vi "Set All Temp (SubVI).vi"(6 "Rate、speed":dbl, 9 "Field输入":dbl, 10 "Approach":i32, 11 "队列输入":refnum<queue>) -> (3 ".NET引用句柄输出":refnum<k24>)   [LabVIEW 2019, in "old.lvlib"]
uses:
  lib/QDInstrument.dll
  config.ctl
  Instrument.ctl
  <vilib>/NI/Modbus Library/API/Master/Modbus Master.lvclass
  old.lvlib
  SubVI.lvlib
panel:
  # "(真是通道1，假是通道2)"
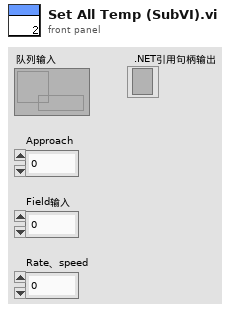
[diagram p1: front panel]
types:
  T1 = typedef "config.ctl" = cluster{"initialize":string, "6221":cluster{"6221 Resource":refnum<visa-resource-name>, "Delta status":bool}, "7001":cluster{"Ch":bool}, "SR830+6221":cluster{"source":u16, "阻抗":dbl, "量程入 4":i32, "量程入 3":i32, "量程入 2":i32, "量程入 1":i32, "电流":dbl, "SR830 2":bool, "SR830 3":bool, "SR830 4":bool, "SR830 1":bool, "VISA 1":refnum<visa-resource-name>, "VISA 2":refnum<visa-resource-name>, "VISA 3":refnum<visa-resource-name>, "VISA 4":refnum<visa-resource-name>, "量程":enum16{"量程每次测量会判定", "量程不变为设定值"}}, "2400":cluster{"2400":bool, "VISA":refnum<visa-resource-name>}, "ch":cluster{"ch str":string, "ch1":bool, "ch2":bool, "布尔":bool}, "error":bool, "数据文件路径":path, "log":cluster{"log路径":path, "log interval":dbl}, "Instrument":T2}
  T2 = typedef "Instrument.ctl" = cluster{"335 Resource":refnum<visa-resource-name>, "Input (0:A)":u16, "Instrument Type":i32, "quantum design":refnum<k24>, "Heater Output (1:1)":u16, "335state":refnum<vi>, "semaphore":T3, "TCP master instance":refnum<class "Modbus Master.lvclass">}
  T3 = typedef "Semaphore RefNum" = refnum<k1>
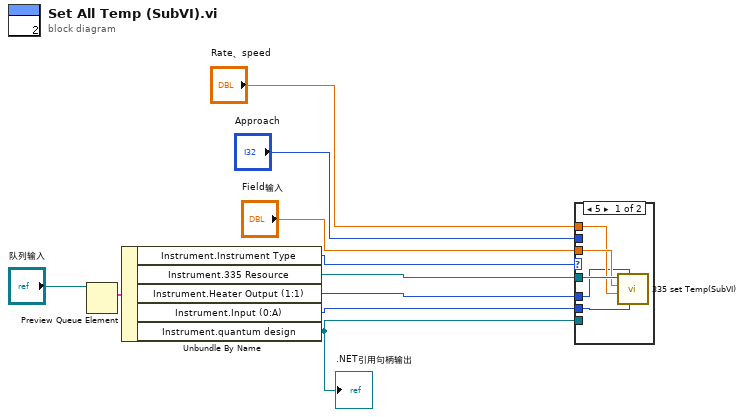
[diagram p0: block diagram]
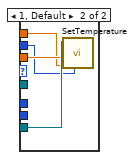
[diagram p2: hidden frame]
diagram:
  n1 = Preview Queue Element(queue="队列输入") -> (element=w5:T1)  [unwired: 2 in, 3 out]
  n2 = Unbundle By Name(w5) -> ("Instrument.Instrument Type"=w10:i32, "Instrument.335 Resource"=w6:refnum<visa-resource-name>, "Instrument.Heater Output (1:1)"=w7:u16, "Instrument.Input (0:A)"=w8:u16, "Instrument.quantum design"=w9:refnum<k24>)
  ".NET引用句柄输出" <- w9
  n3 = case shown="5" w10 {
    tunnel: w9 -> [_ w19]
    tunnel: "Field输入" -> [w14 w18]
    tunnel: "Rate、speed" -> [w13 w17]
    tunnel: "Approach" -> [_ w16]
    tunnel: w6 -> [w15 _]
    tunnel: w7 -> [w12 _]
    tunnel: w8 -> [w11 _]
    frame 5 {
      n4 = call "335 set Temp(SubVI).vi"("Input (0:A)"=w11, "Output (1:1)"=w12, "Rate"=w13, "Temperature"=w14, "VISA Refnum in"=w15) -> ()  [unwired: 5 in, 2 out]
    }
    frame 1, Default {
      n5 = call "SetTemperature.vi"("Approach"=w16, "Rate"=w17, "Temperature"=w18, "Instrument Ref In"=w19) -> ()  [unwired: 3 in, 3 out]
    }
  }
